vi "read_file.vi"() -> ()   [LabVIEW 2015]
panel:
  out "error out":errorcluster
  out "Last line read":string
  in  "File to read":path
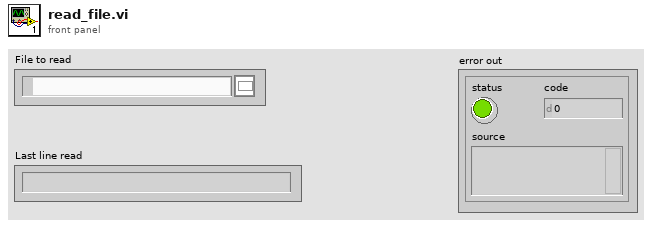
[diagram p1: front panel]
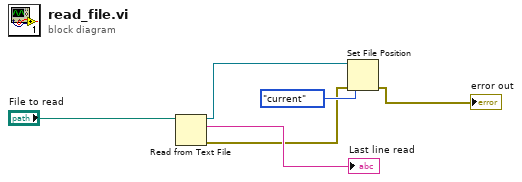
[diagram p0: block diagram]
diagram:
  n1 = Read from Text File(file (use dialog)="File to read") -> (refnum out=w3:refnum<file>, text=→"Last line read":string, error out=w1:errorcluster)  [unwired: 3 in, 1 out]
  n2 = Set File Position(refnum=w3, from (0:start)=enum16{"start", "end", "current"}."current", error in=w1) -> (error out=→"error out":errorcluster)  [unwired: 1 in, 1 out]
